vi "GV DO7.vi"() -> ()   [LabVIEW 2017]
panel:
  out "DO7":bool
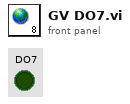
[diagram p1: front panel]
diagram:
